vi "ReadAll_5772.vi"(9 "# elements to keep in DMA":u32, 11 "scope params":T1={"scope mode"=enum."Stopped", "ticker"=refnum, "5160 samples per trigger"=0, "FPGA ref"=refnum, "P2P params"={"instrument handle"="", "stream session"=refnum, "scale"={"offset"=0.0, "gain"=0.0, "reserved 1"=0.0, "reserved 2"=0.0}, "actual sample rate"=10000000.0, "Trigger"=enum."PFI 0", "SCOPE Resource"="Dev1", "input impedance"=0}, "data mode"=enum."Real IO", "5782 samples per record"=0, "Chart length"=0} {"P2P params"."input impedance" items=["1 mega ohm"=0, "50 ohms"=2]; "P2P params"."actual sample rate" format="%.2p"}) -> (1 "Data":u64[](array[numeric]), 3 "scope params":T1={"scope mode"=enum."Stopped", "ticker"=refnum, "5160 samples per trigger"=0, "FPGA ref"=refnum, "P2P params"={"instrument handle"="", "stream session"=refnum, "scale"={"offset"=0.0, "gain"=0.0, "reserved 1"=0.0, "reserved 2"=0.0}, "actual sample rate"=10000000.0, "Trigger"=enum."PFI 0", "SCOPE Resource"="Dev1", "input impedance"=0}, "data mode"=enum."Real IO", "5782 samples per record"=0, "Chart length"=0} {"P2P params"."input impedance" items=["1 mega ohm"=0, "50 ohms"=2]; "P2P params"."actual sample rate" format="%.2p"})   [LabVIEW 2013]
uses:
  <vilib>/rvi/interface/nirviMethod/nirviMethod.xnode
  <vilib>/FPGAPlugInAG/Dynamic/niLvFpga_ReadFifo_Dynamic.vi
  <vilib>/rvi/errors/niLvFpgaMergeErrorWithErrorCode.vi
  Config/FPGAref.ctl
  controls/ScopeMode.ctl
  Utilities/Ticker/Ticker.lvclass
  trigger_source.ctl
  P2P params.ctl
  FPGA/DataMode.ctl
  controls/scope_params.ctl
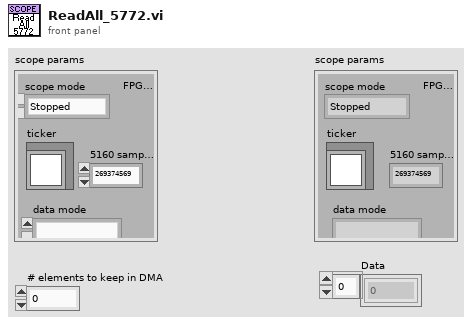
[diagram p1: front panel]
types:
  T1 = typedef "scope_params.ctl" = cluster{"scope mode":T2, "ticker":refnum<class "Ticker.lvclass">, "5160 samples per trigger":u32, "FPGA ref":T3, "P2P params":T4, "data mode":T6, "5782 samples per record":u32, "Chart length":i32}
  T2 = typedef "ScopeMode.ctl" = enum16{"Stopped", "Single", "Running", "Continuous"}
  T3 = typedef "FPGAref.ctl" = refnum<k20>
  T4 = typedef "P2P params.ctl" = cluster{"instrument handle":refnum<k15>, "stream session":refnum<k20>, "scale":cluster{"offset":dbl, "gain":dbl, "reserved 1":dbl, "reserved 2":dbl}, "actual sample rate":dbl, "Trigger":T5, "SCOPE Resource":refnum<k15>, "input impedance":u32}
  T5 = typedef "trigger_source.ctl" = enum16{"PFI 0", "PFI 1", "Software"}
  T6 = typedef "DataMode.ctl" = enum16{"Real IO", "Simulated"}
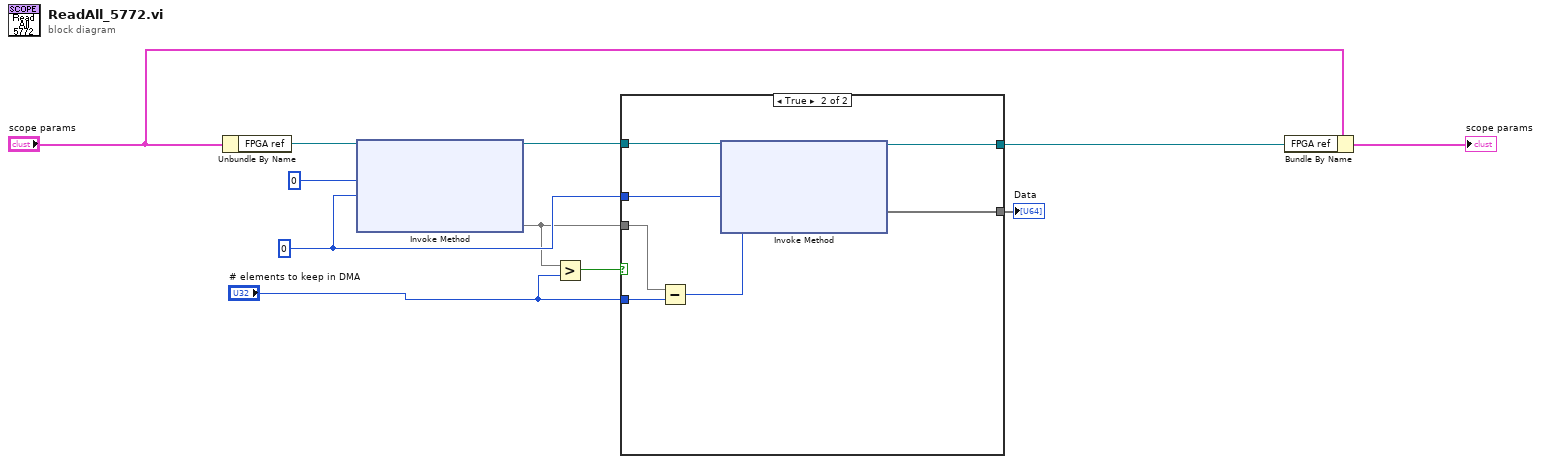
[diagram p0: block diagram]
diagram:
  w8 = 0 ("Timeout (ms)")
  n1 = Unbundle By Name("scope params") -> ("FPGA ref"=w11:T3)
  n2 = xnode "Invoke Method"("FPGA VI Reference In"=w11, "Number of Elements"=u32 0, "Timeout (ms)"=w8) -> ("FPGA VI Reference Out"=w9:T3, "Elements Remaining"=w5)  [unwired: 1 in, 2 out]
  n3 = Greater?(x=w5, y="# elements to keep in DMA") -> (0:w3:bool)
  n4 = case shown="True" w3 {
    tunnel: w9 -> [w12 w19]
    tunnel: w8 -> [_ w18]
    tunnel: w5 -> [_ w16]
    tunnel: "# elements to keep in DMA" -> [_ w17]
    tunnel: [_ w14] -> w2
    tunnel: [w12 w13] -> w1
    frame False {
    }
    frame True {
      n5 = Subtract(x=w16, y=w17) -> (x-y=w15:u32)
      n6 = xnode "Invoke Method"("FPGA VI Reference In"=w19, "Number of Elements"=w15, "Timeout (ms)"=w18) -> ("FPGA VI Reference Out"=w13:T3, "Data"=w14:void[])  [unwired: 1 in, 2 out]
    }
  }
  "Data" <- w2
  n7 = Bundle By Name(cluster="scope params", "FPGA ref"=w1) -> (→"scope params":T1)
